vi "MILStateFeedbackControllerXY.vi"(0 "Ac":dbl[](array[numeric])=[0.0, 0.0, 0.0, 0.0], 1 "DispX":dbl, 3 "P1X":dbl, 6 "DispY":dbl, 7 "Bc":dbl[](array[numeric])=[0.0, 0.0, 0.0, 0.0], 9 "Cc":dbl[](array[numeric])=[1.0, 0.0], 10 "ForceY":dbl, 11 "Dc":dbl[](array[numeric])=[0.0, 0.0], 12 "ForceX":dbl, 14 "P2X":dbl) -> (4 "ValveCMDX":dbl, 8 "StateX":dbl[](array[numeric]), 13 "StateY":dbl[](array[numeric]), 15 "ValveCMDY":dbl)   [LabVIEW 2020]
uses:
  <vilib>/Analysis/NI_AALBase.lvlib
  <vilib>/Analysis/baseanly.llb/A x Vector.vi
  <vilib>/Analysis/NI_AALBLAS.lvlib
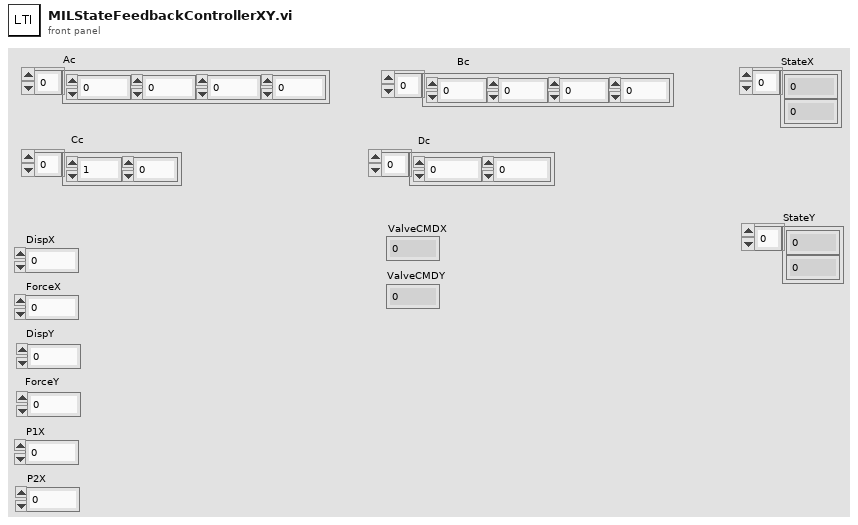
[diagram p1: front panel]
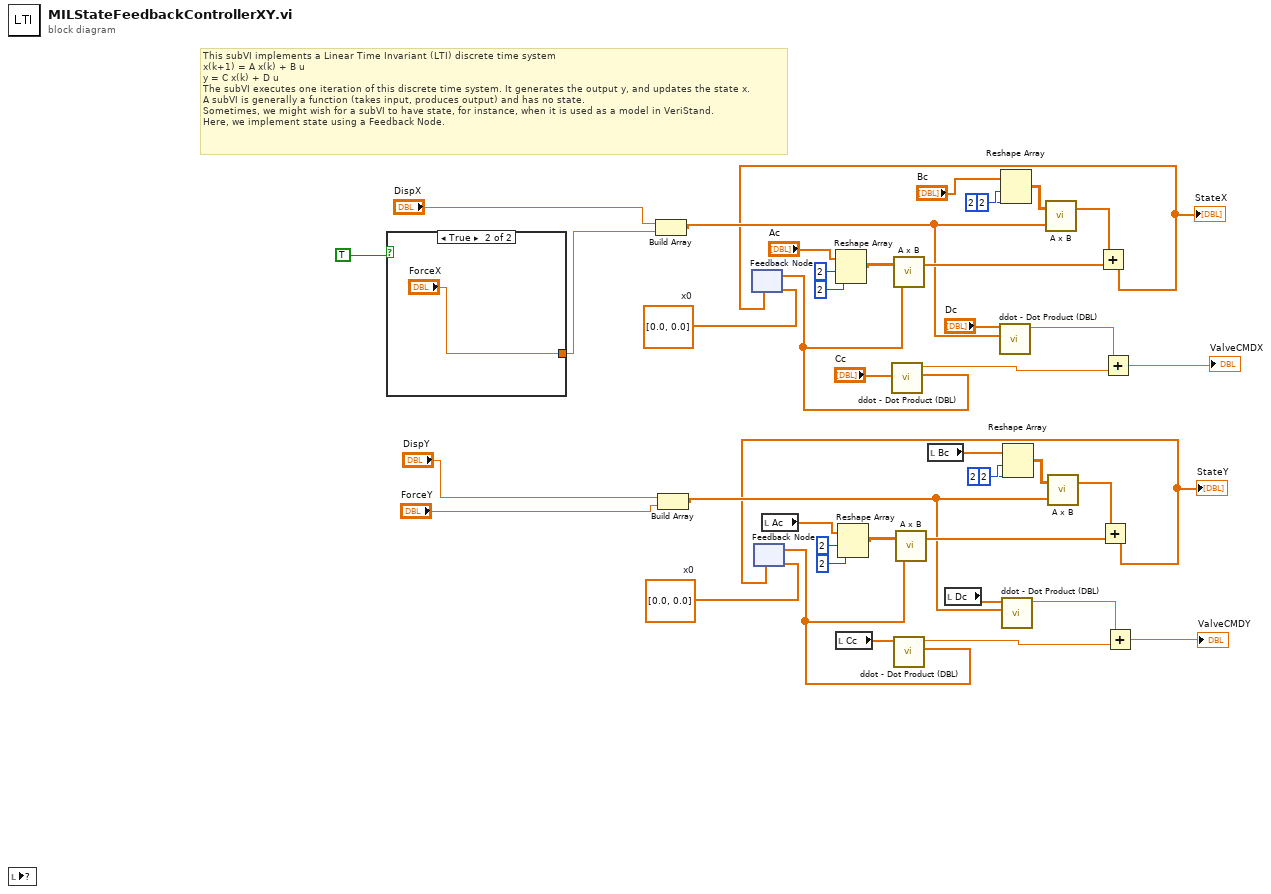
[diagram p0: block diagram]
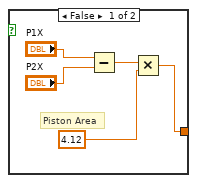
[diagram p2: hidden frame]
diagram:
  w21 = dbl[] [0.0, 0.0]  # x0
  w43 = dbl[] [0.0, 0.0]  # x0
  # "This subVI implements a Linear Time Invariant (LTI) discrete time system\nx(k+1) = A x(k) + B u\ny = C x(k) + D u\nThe subVI executes one iteration of this discrete time system. It generates the output y, and updates the state x.\nA subVI is generally a function (takes input, produces output) and has no state.\nSometimes, we might wish for a subVI to have state, for instance, when it is used as a model in VeriStand.\nHere, we implement state using a Feedback Node."
  n1 = local read item#-1() -> ()  [unwired: 1 in]
  n2 = case shown="True" TRUE {
    tunnel: [w44 "ForceX"] -> w33
    frame False {
      # "Piston Area"
      n3 = Subtract(x="P1X", y="P2X") -> (x-y=w48:dbl)
      n4 = Multiply(x=w48, y=4.12) -> (x*y=w44:dbl)
    }
    frame True {
    }
  }
  n5 = Build Array("DispX", w33) -> (w32:dbl[])
  n6 = Build Array("DispY", "ForceY") -> (w15:dbl[])
  n7 = feedback #1(w43) -> (w41:dbl[])
  n8 = feedback #2(w21) -> (w19:dbl[])
  n9 = local read "Ac"() -> (w7:dbl[])
  n10 = Reshape Array("Ac", 2 ("dimension size"), 2 ("dimension size")) -> (w28:dbl[][])
  n11 = local read "Cc"() -> (w2:dbl[])
  n12 = Reshape Array(w7, 2 ("dimension size"), 2 ("dimension size")) -> (w12:dbl[][])
  n13 = call <vilib>:"ddot - Dot Product (DBL).vi"("y"=w41, "x"="Cc") -> ("ddot"=w40:dbl)  [unwired: 8 in, 1 out]
  n14 = call-poly <vilib>:"A x B.vi"("Vector"=w41, "A"=w28) -> ("A x Vector"=w42:dbl[])  [unwired: 1 out]
  n15 = call <vilib>:"ddot - Dot Product (DBL).vi"("y"=w19, "x"=w2) -> ("ddot"=w18:dbl)  [unwired: 8 in, 1 out]
  n16 = call-poly <vilib>:"A x B.vi"("Vector"=w19, "A"=w12) -> ("A x Vector"=w20:dbl[])  [unwired: 1 out]
  n17 = local read "Bc"() -> (w6:dbl[])
  n18 = local read "Dc"() -> (w3:dbl[])
  n19 = call <vilib>:"ddot - Dot Product (DBL).vi"("y"=w32, "x"="Dc") -> ("ddot"=w37:dbl)  [unwired: 8 in, 1 out]
  n20 = Reshape Array("Bc", 2 ("dimension size"), 2 ("dimension size")) -> (w24:dbl[][])
  n21 = call <vilib>:"ddot - Dot Product (DBL).vi"("y"=w15, "x"=w3) -> ("ddot"=w16:dbl)  [unwired: 8 in, 1 out]
  n22 = Reshape Array(w6, 2 ("dimension size"), 2 ("dimension size")) -> (w9:dbl[][])
  n23 = call-poly <vilib>:"A x B.vi"("Vector"=w32, "A"=w24) -> ("A x Vector"=w39:dbl[])  [unwired: 1 out]
  n24 = call-poly <vilib>:"A x B.vi"("Vector"=w15, "A"=w9) -> ("A x Vector"=w17:dbl[])  [unwired: 1 out]
  n25 = Add(x=w39, y=w42) -> (x+y=w22:dbl[])
  "StateX" <- w22
  n26 = feedback-in #1(w22) -> ()
  n27 = Add ("Add.vi")(x=w17, y=w20) -> (x+y=w8:dbl[])
  "StateY" <- w8
  n28 = feedback-in #2(w8) -> ()
  n29 = Add(x=w37, y=w40) -> (x+y=→"ValveCMDX":dbl)
  n30 = Add(x=w16, y=w18) -> (x+y=→"ValveCMDY":dbl)
